vi "Main.vi"() -> ()   [LabVIEW 2021]
doc: "This template is for the Queued Message Handler design pattern.\n\nThe Event Handling Loop generates messages based on user interface actions.\n\nThe Message Handling Loop processes messages generated by the Event Handling Loop, or by other messages. The messages are string values, so new messages can be added easily to the Message Cases case structure in the Message Handling Loop. Each message cluster can also provide an optional value for Message Data, which is a variant that can be converted to whatever message-specific data is required."
uses:
  Czytaj RS/Biblioteki/Statyw/Sending Params.ctl
  controls/UI Data.ctl
  controls/STAV Data.ctl
  Czytaj RS/Biblioteki/Statyw/STAV CommandList.ctl
  support/Message Queue/Enqueue Message (Single).vi
  <vilib>/Utility/error.llb/Error Cluster From Error Code.vi
  <vilib>/ErrorRing/Error Ring.xnode
  support/Message Queue/Message Queue.lvlib
  support/User Event - Stop/User Event - Stop.lvlib
  Czytaj RS/Biblioteki/Statyw/STAV lib.lvlib
panel:
  out "str command":string
  out "String 2":string
  out "String":string
  out "Display <Replace Me>":string
  in  "Exit":bool
  in  "Tab Control":T1(tab)
  in  "STAV com port":refnum<visa-resource-name>="COM6"
  in  "Sending Params (set before RUN)":T2={"[s]peed"=FALSE, "[p]osition"=TRUE, "[f]orce"=TRUE, "p[e]ak force"=FALSE, "pe[a]k distance"=FALSE, "[t]ravel"=FALSE, "[m]s"=TRUE, "[c]ycle no"=FALSE, "step [n]o"=FALSE, "[d]uration"=FALSE, "p[r]ofile position"=FALSE, "[h]old time"=FALSE}
  in  "Sending Interval":i32=500 min=1 max=10000 step=1
  in  "StopSending":bool
  in  "Velocity":i32=30
  in  "Position":dbl
  in  "HomePos":bool
  in  "Start Sending":bool
  in  "Clear 2":bool
  out "Log 2":string
  in  "Clear":bool
  out "Log":string
  in  "Do Something <Replace Me>":bool
  in  "Do Something Else <Replace Me>":bool
  # "These controls have associated \"Value Changed\" events configured in the Event Structure on the diagram.\n\nReplace them (and reconfigure the Event Structure) with the controls you need for your application."
  # "This template is for the Queued Message Handler design pattern.\n\nSee the block diagram for more information on how to use this template."
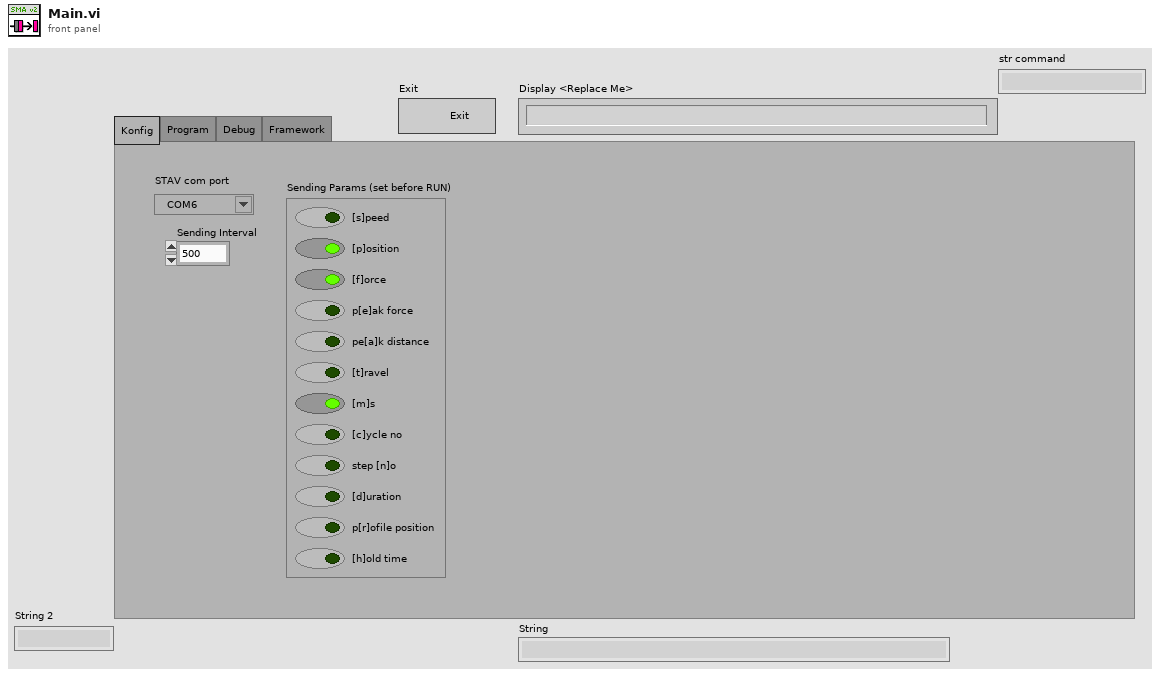
[diagram p1: front panel]
types:
  T1 = enum32{"Konfig", "Program", "Debug", "Framework"}
  T2 = typedef "STAV lib.lvlib/Sending Params.ctl" = cluster{"[s]peed":bool, "[p]osition":bool, "[f]orce":bool, "p[e]ak force":bool, "pe[a]k distance":bool, "[t]ravel":bool, "[m]s":bool, "[c]ycle no":bool, "step [n]o":bool, "[d]uration":bool, "p[r]ofile position":bool, "[h]old time":bool}
  T3 = typedef "STAV Data.ctl" = cluster{"STAV ref":refnum<visa-resource-name>}
  T4 = typedef "UI Data.ctl" = cluster{"Boolean <Replace Me>":bool, "String <Replace Me>":string, "Numeric <Replace Me>":dbl, "Do Something Ref":refnum<vi>, "Do Something Else Ref":refnum<vi>, "Data Display Ref":refnum<vi>, "Exit Button Ref":refnum<vi>}
  T5 = typedef "Message Queue.lvlib/All Message Queues.ctl" = cluster{"UI":refnum<queue>, "Display":refnum<queue>, "Stav":refnum<queue>, "DAQ":refnum<queue>}
  T6 = typedef "STAV lib.lvlib/STAV CommandList.ctl" = enum16{"StartSending (0)", "StopSending(0)", "FindHomePos(0)", "SetSendingConfig(2)", "GetSendingConfig(0)", "SetPosition(2)", "SetSpeed(2)", "GetSpeed(0)", "GetPosition(0)", "GetForce(0)", "GetPeak(0)", "GetPeakDistance(0)", "GetTravelDistance(0)", "ResetTravelDistance(0)", "GetCycleNo(0)", "GetStepNo(0)", "GetDuration(0)", "GetProfilePosition(0)", "GetHoldTime(0)", "Stop(0)", "StartAndSend(0)", "Start(0)", "Reset(0)", "GetActiveProfile(0)", "SetActiveProfile(2)", "GetProfileCnt(1)", "GetMaxStepCnt(1)", "GetStepCnt(2)", "GetProfileIndex(2)", "SetProfile(3)", "SetStep(3+params)", "GetProfile(2)", "GetStep(3)", "SetProfile(2+params)", ""}
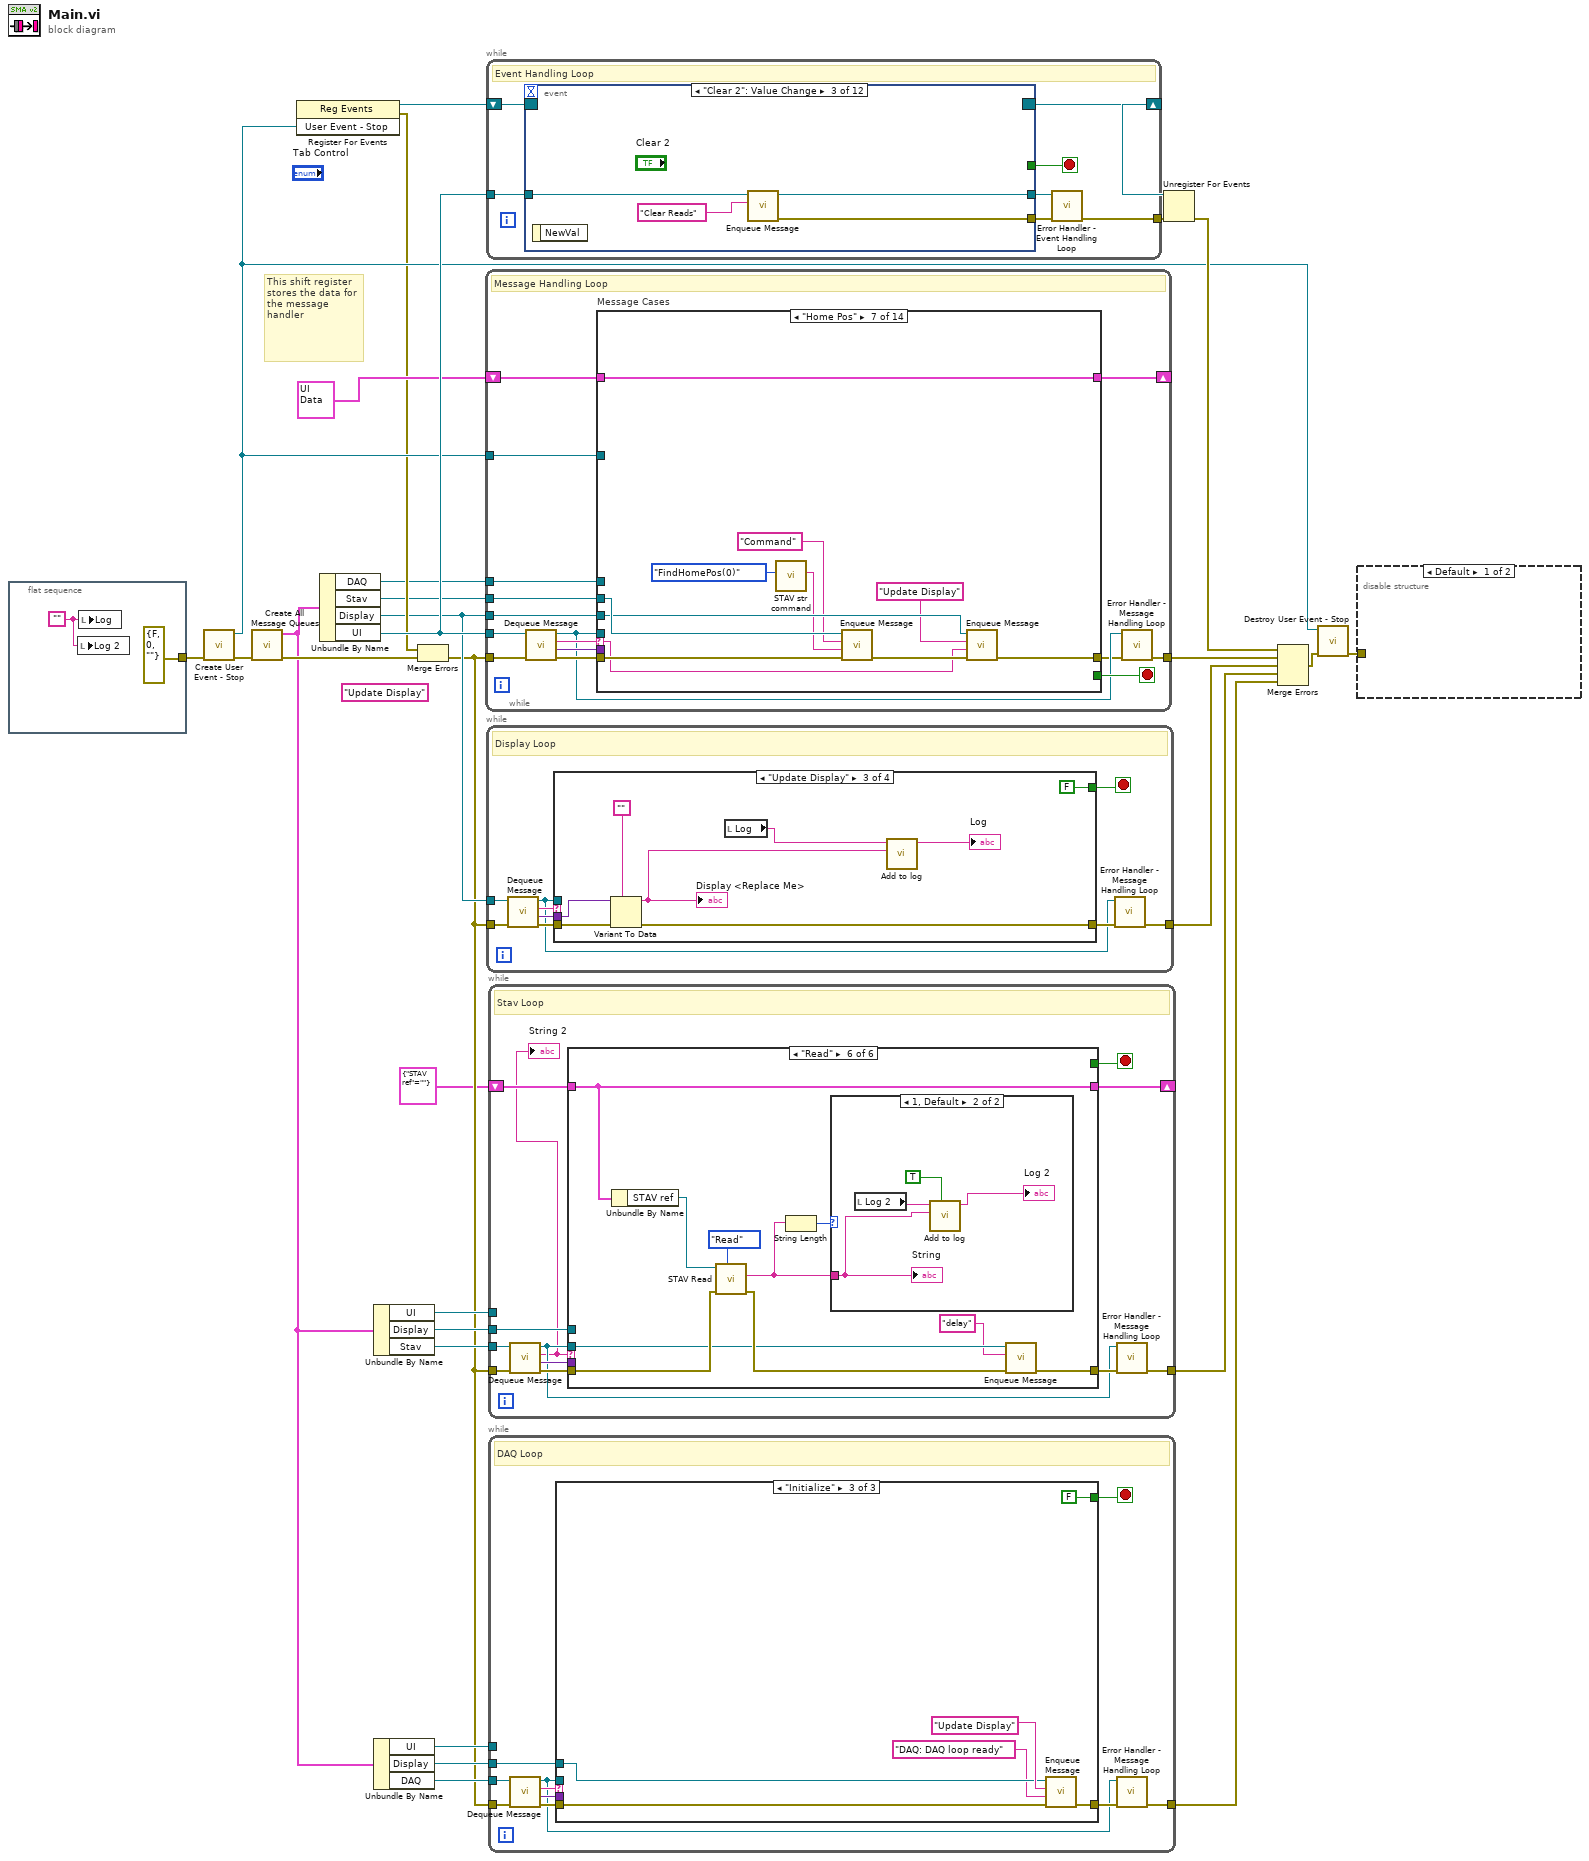
[diagram p0: block diagram]
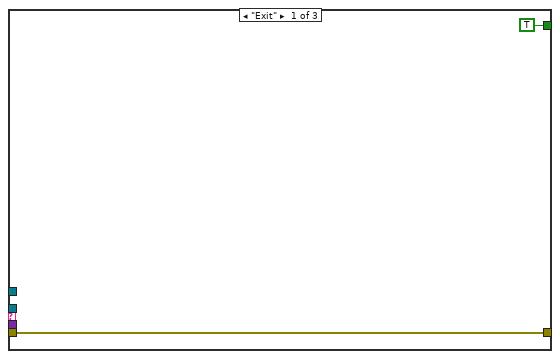
[diagram p2: hidden frame]
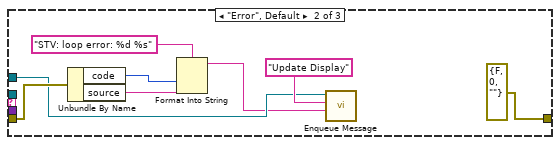
[diagram p3: hidden frame]
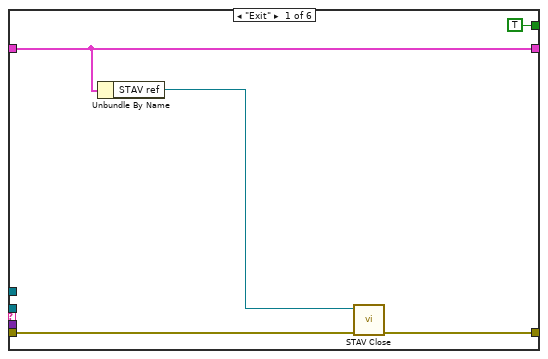
[diagram p4: hidden frame]
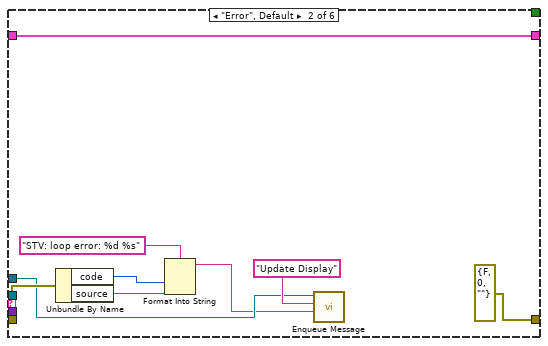
[diagram p5: hidden frame]
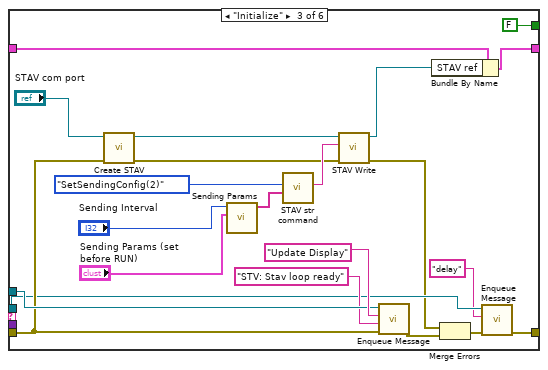
[diagram p6: hidden frame]
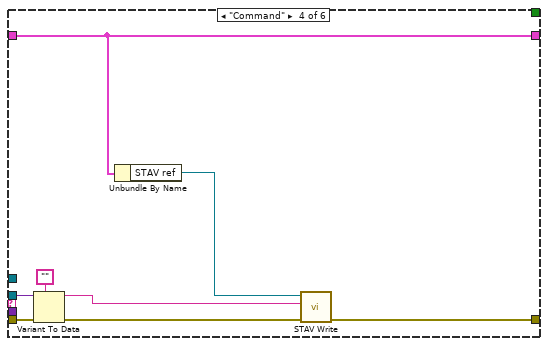
[diagram p7: hidden frame]
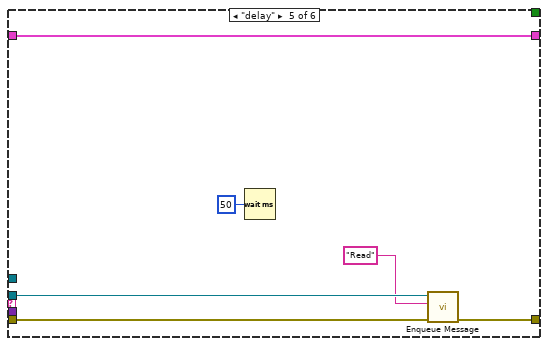
[diagram p8: hidden frame]
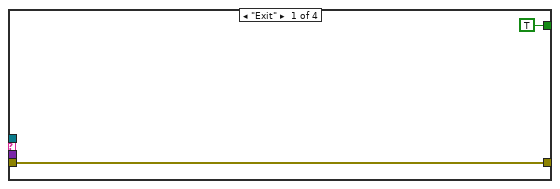
[diagram p10: hidden frame]
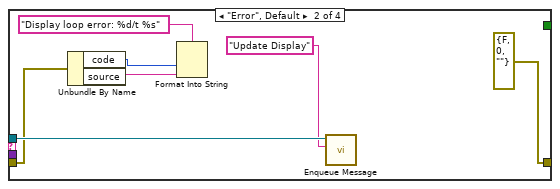
[diagram p11: hidden frame]
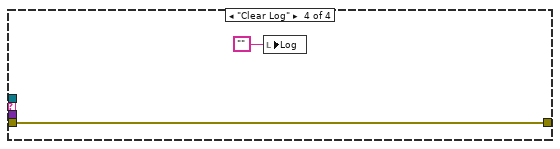
[diagram p12: hidden frame]
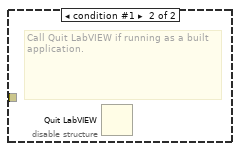
[diagram p13: hidden frame]
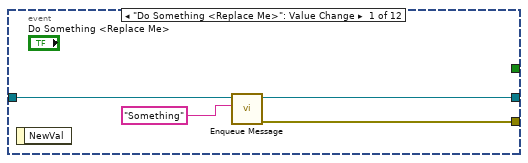
[diagram p14: hidden frame]
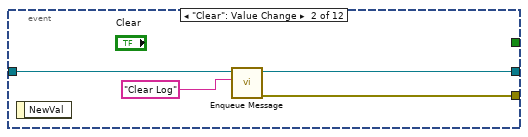
[diagram p15: hidden frame]
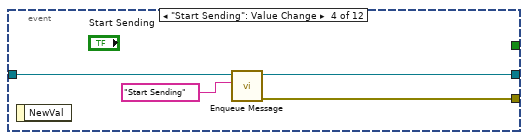
[diagram p16: hidden frame]
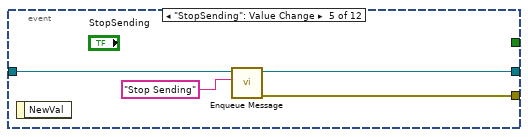
[diagram p17: hidden frame]
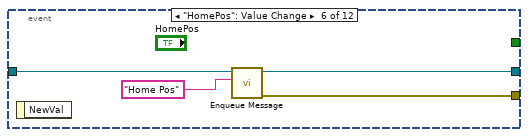
[diagram p18: hidden frame]
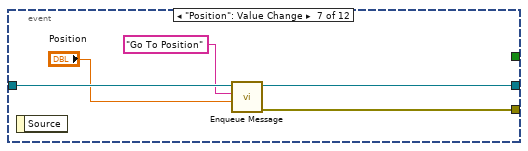
[diagram p19: hidden frame]
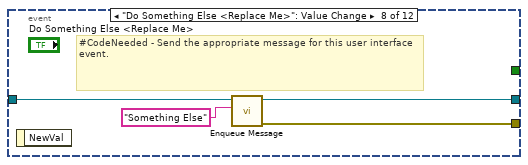
[diagram p20: hidden frame]
diagram:
  (unwired) "Update Display" ("Message")
  # "This shift register stores the data for the message handler"
  n1 = flat-sequence {
    tunnel: [errorcluster {"status"=FALSE, "code"=0, "source"=""} ("error constant")] -> w11
    frame #0 {
      w30 = ""
      n2 = local write "Log 2"(w30) -> ()
      n3 = local write "Log"(w30) -> ()
    }
  }
  n4 = call "Create User Event - Stop.vi"("error in (no error)"=w11) -> ("error out"=w26:errorcluster, "User Event - Stop"=w18:refnum<user-event>)  [unwired: 9 in]
  n5 = call "Create All Message Queues.vi"("error in (no error)"=w26) -> ("error out"=w29:errorcluster, "Message Queues out"=w4:T5)  [unwired: 9 in]
  n6 = register-events(w18) -> (reference out=w19:refnum<event-registration>, error out=w17:errorcluster)  [unwired: 2 in]
  n7 = Unbundle By Name(w4) -> ("DAQ"=w14:refnum<queue>, "Stav"=w15:refnum<queue>, "Display"=w16:refnum<queue>, "UI"=w27:refnum<queue>)
  n8 = Unbundle By Name(w4) -> ("UI"=w8:refnum<queue>, "Display"=w12:refnum<queue>, "Stav"=w13:refnum<queue>)
  n9 = Unbundle By Name(w4) -> ("UI"=w7:refnum<queue>, "Display"=w6:refnum<queue>, "DAQ"=w5:refnum<queue>)
  n10 = Merge Errors(w17, w29) -> (w2:errorcluster)
  n11 = while {
    tunnel: w27 -> [w38]
    shift-right: [w45] -> _
    shift-left: T4 {"Boolean <Replace Me>"=FALSE, "String <Replace Me>"="", "Numeric <Replace Me>"=0.0, "Do Something Ref"=refnum, "Do Something Else Ref"=refnum, "Data Display Ref"=refnum, "Exit Button Ref"=refnum} ("Data Cluster") -> [w46]
    tunnel: w18 -> [w43]
    tunnel: w2 -> [w42]
    tunnel: [w36] -> w28
    tunnel: w16 -> [w34]
    tunnel: w15 -> [w33]
    tunnel: w14 -> [w32]
    stop <- w44 stop-if-true
    # "Message Handling Loop"
    n12 = call "Dequeue Message.vi"("error in (no error)"=w42, "Message Queue"=w38) -> ("error out"=w41:errorcluster, "Message Data"=w39:variant, "Message"=w40:string, "dup Message Queue"=w37:refnum<queue>)  [unwired: 6 in]
    n13 = case "Message Cases" shown="\"Home Pos\"" w40 {
      selector: w40 -> [_ _ _ _ w81 w92 w103 w121 w129 _ _ _ w151 w171]
      tunnel: w37 -> [_ _ _ _ _ _ _ _ _ _ w142 _ w170 _]
      tunnel: w41 -> [w55 w61 w68 w77 w87 w98 w109 w115 w131 w138 w146 w149 w164 _]
      tunnel: [w56 w62 w69 w71 w84 w95 w106 w124 w130 w137 w144 w147 w167 w172] -> w35
      tunnel: w46 -> [w54 w63 w70 w76 w88 w99 w110 w127 w132 w139 w145 w148 w169 w173]
      tunnel: [w53 w63 w70 w76 w88 w99 w110 w127 w132 w139 w145 w148 w169 w173] -> w45
      tunnel: [_ _ _ _ _ _ _ _ _ _ _ _ TRUE _] -> w44
      tunnel: w39 -> [_ _ _ w75 _ _ _ w113 _ _ _ _ w161 _]
      tunnel: w43 -> [_ _ _ _ _ _ _ _ _ _ _ _ w166 _]
      tunnel: w34 -> [w47 w57 w64 _ w83 w94 w105 w123 w128 w136 _ _ w159 _]
      tunnel: w33 -> [_ _ _ _ w86 w97 w108 w126 _ _ _ _ w154 _]
      tunnel: w32 -> [_ _ _ _ _ _ _ _ _ _ _ _ w150 _]
      frame "Initialize" {
        w50 = "MHL: Program Ready" ("Initial Message")
        # "Initialize - All initialization work should take place in this message, since other loops can potentially enqueue messages that execute immediately after this one."
        n14 = control-ref of="Do Something <Replace Me>"() -> (w48:refnum<vi>)
        n15 = control-ref of="Do Something Else <Replace Me>"() -> (w49:refnum<vi>)
        n16 = control-ref of="Exit"() -> (w52:refnum<vi>)
        n17 = Bundle By Name(cluster=w54, "Do Something Ref"=w48, "Do Something Else Ref"=w49, "Exit Button Ref"=w52, "String <Replace Me>"=w50) -> (w53:T4)
        n18 = call-poly "Enqueue Message.vi"("error in (no error)"=w55, "Message Data"=w50, "Message"="Update Display", "Message Queue"=w47) -> ("error out"=w56:errorcluster)  [unwired: 6 in, 1 out]
      }
      frame "Something" {
        # "Send string to \"Update Display\" message"
        # "#CodeNeeded - Perform whatever actions correspond to the \"Something\" message."
        # "Something - Replace this message with functionality for your own application."
        n19 = call-poly "Enqueue Message.vi"("error in (no error)"=w61, "Message Data"="\"Do Something\" button pressed" ("\"Do Something\" button pressed"), "Message"="Update Display", "Message Queue"=w57) -> ("error out"=w60:errorcluster)  [unwired: 6 in, 1 out]
        n20 = Merge Errors(w60) -> (w62:errorcluster)
      }
      frame "Something Else" {
        # "Send string to \"Update Display\" message"
        # "#CodeNeeded - Perform whatever actions correspond to the \"Something Else\" message."
        # "Something Else - Replace this message with functionality for your own application."
        n21 = call-poly "Enqueue Message.vi"("error in (no error)"=w68, "Message Data"="\"Do Something Else\" button pressed" ("\"Do Something Else\" button pressed"), "Message"="Update Display", "Message Queue"=w64) -> ("error out"=w67:errorcluster)  [unwired: 6 in, 1 out]
        n22 = Merge Errors(w67) -> (w69:errorcluster)
      }
      frame "Error" {
        # "#CodeRecommended - If you ever change the name of this \"Error\" message, you'll need to update the name in the Check Loop Error.vi as well."
        # "#CodeRecommended - Consider creating a system for logging errors in some way. These errors are for notification purposes only. Handling of specific errors should be performed in the message frames that generated the error."
        # "Error - Display an error dialog. This message is sent by the \"Error Handler\" VIs at the end of other loops in this application."
        n23 = Variant To Data(error in=w77, type=errorcluster {"status"=FALSE, "code"=0, "source"=""} ("error constant"), Variant=w75) -> (data=w73:errorcluster, error out=w72:errorcluster)
        n24 = call <vilib>:"Simple Error Handler.vi"("error in (no error)"=w73) -> ()  [unwired: 4 in, 5 out]
        n25 = Merge Errors(w72) -> (w71:errorcluster)
      }
      frame "Start Sending" {
        n26 = call "STAV str command.vi"("Command"=STAV_CommandList."StartSending (0)") -> ("str command"=w79:string)  [unwired: 9 in, 1 out]
        n27 = call-poly "Enqueue Message.vi"("error in (no error)"=w87, "Message Data"=w79, "Message"="Command", "Message Queue"=w86) -> ("error out"=w85:errorcluster)  [unwired: 6 in, 1 out]
        n28 = call-poly "Enqueue Message.vi"("error in (no error)"=w85, "Message Data"=w81, "Message"="Update Display", "Message Queue"=w83) -> ("error out"=w84:errorcluster)  [unwired: 6 in, 1 out]
      }
      frame "Stop Sending" {
        n29 = call "STAV str command.vi"("Command"=STAV_CommandList."StopSending(0)") -> ("str command"=w90:string)  [unwired: 9 in, 1 out]
        n30 = call-poly "Enqueue Message.vi"("error in (no error)"=w98, "Message Data"=w90, "Message"="Command", "Message Queue"=w97) -> ("error out"=w96:errorcluster)  [unwired: 6 in, 1 out]
        n31 = call-poly "Enqueue Message.vi"("error in (no error)"=w96, "Message Data"=w92, "Message"="Update Display", "Message Queue"=w94) -> ("error out"=w95:errorcluster)  [unwired: 6 in, 1 out]
      }
      frame "Home Pos" {
        n32 = call "STAV str command.vi"("Command"=STAV_CommandList."FindHomePos(0)") -> ("str command"=w101:string)  [unwired: 9 in, 1 out]
        n33 = call-poly "Enqueue Message.vi"("error in (no error)"=w109, "Message Data"=w101, "Message"="Command", "Message Queue"=w108) -> ("error out"=w107:errorcluster)  [unwired: 6 in, 1 out]
        n34 = call-poly "Enqueue Message.vi"("error in (no error)"=w107, "Message Data"=w103, "Message"="Update Display", "Message Queue"=w105) -> ("error out"=w106:errorcluster)  [unwired: 6 in, 1 out]
      }
      frame "Go To Position" {
        n35 = Variant To Data(error in=w115, type=0.0, Variant=w113) -> (data=w111:dbl, error out=w114:errorcluster)
        n36 = call "Position Attributes.vi"("Speed"="Velocity", "Position"=w111) -> ("array"=w117:string[])  [unwired: 8 in, 1 out]
        n37 = call "STAV str command.vi"("Params"=w117, "Command"=STAV_CommandList."SetPosition(2)") -> ("str command"=w119:string)  [unwired: 8 in, 1 out]
        "str command" <- w119
        n38 = call-poly "Enqueue Message.vi"("error in (no error)"=w114, "Message Data"=w119, "Message"="Command", "Message Queue"=w126) -> ("error out"=w125:errorcluster)  [unwired: 6 in, 1 out]
        n39 = call-poly "Enqueue Message.vi"("error in (no error)"=w125, "Message Data"=w121, "Message"="Update Display", "Message Queue"=w123) -> ("error out"=w124:errorcluster)  [unwired: 6 in, 1 out]
      }
      frame "Clear Log" {
        n40 = call-poly "Enqueue Message.vi"("error in (no error)"=w131, "Message"=w129, "Message Queue"=w128) -> ("error out"=w130:errorcluster)  [unwired: 7 in, 1 out]
      }
      frame "Clear Reads" {
        n41 = call-poly "Enqueue Message.vi"("error in (no error)"=w138, "Message Data"="MHL: Clear Reads" ("Message"), "Message"="Update Display", "Message Queue"=w136) -> ("error out"=w137:errorcluster)  [unwired: 6 in, 1 out]
        n42 = local write "Log 2"("") -> ()
      }
      frame "Confirm Quit" {
        # "#CodeNeeded - If you want to provide an \"Are you sure\" dialog (or some other notification) before the application exits, place that code here. This message is typically sent from a Panel Close? event."
        # "Confirm Quit - Message that can confirm whether or not the user wants to exit the application."
        n43 = call-poly "Enqueue Message.vi"("Priority Message? (F)"=TRUE, "error in (no error)"=w146, "Message"="Exit", "Message Queue"=w142) -> ("error out"=w143:errorcluster)  [unwired: 6 in, 1 out]
        n44 = Merge Errors(w143) -> (w144:errorcluster)
      }
      frame "---Copy This Frame---" {
        # "Duplicate this frame when creating new messages.  Change this comment in the duplicated frame to describe this message."
        n45 = Merge Errors(w149) -> (w147:errorcluster)
      }
      frame "Exit" {
        # "Stop the VI"
        # "#CodeNeeded - Add any required cleanup code here. Note that if 'Exit' was called as a result of an error, an error dialog will be displayed. Add any custom error handling for an 'Exit' condition here as well."
        # "Exit - Exit the application."
        n46 = Variant To Data(type=errorcluster {"status"=FALSE, "code"=0, "source"=""} ("error constant"), Variant=w161) -> (data=w162:errorcluster)  [unwired: 1 in, 1 out]
        n47 = Release Queue(queue=w170, error in (no error)=w164) -> (error out=w160:errorcluster)  [unwired: 1 in, 2 out]
        n48 = call <vilib>:"Simple Error Handler.vi"("error in (no error)"=w162) -> ()  [unwired: 4 in, 5 out]
        n49 = call-poly "Enqueue Message.vi"("error in (no error)"=w160, "Message Data"=w151, "Message"="Update Display", "Message Queue"=w159) -> ("error out"=w156:errorcluster, "dup Message Queue"=w157:refnum<queue>)  [unwired: 6 in]
        n50 = call-poly "Enqueue Message.vi"("error in (no error)"=w156, "Message"=w151, "Message Queue"=w157) -> ("error out"=w155:errorcluster)  [unwired: 7 in, 1 out]
        n51 = call "Fire User Event - Stop.vi"("User Event - Stop"=w166) -> ("error out"=w165:errorcluster)  [unwired: 10 in]
        n52 = call-poly "Enqueue Message.vi"("error in (no error)"=w155, "Message"=w151, "Message Queue"=w154) -> ("error out"=w153:errorcluster)  [unwired: 7 in, 1 out]
        n53 = call-poly "Enqueue Message.vi"("error in (no error)"=w153, "Message"=w151, "Message Queue"=w150) -> ("error out"=w152:errorcluster)  [unwired: 7 in, 1 out]
        n54 = Merge Errors(w165, w152) -> (w167:errorcluster)
      }
      frame Default {
        # "'Default' case only runs if there is a message that isn't defined in any of the other cases.  Output a programming error."
        n55 = xnode "Error Ring"("parameter 0"=w171) -> ("error out"=w172:errorcluster)
      }
    }
    n56 = call "Error Handler - Message Handling Loop.vi"("error in (no error)"=w35, "Message Queue"=w37) -> ("dup error in"=w36:errorcluster)  [unwired: 8 in, 1 out]
  }
  n57 = while {
    tunnel: w27 -> [w187]
    shift-right: [w185] -> w23
    shift-left: w19 -> [w186]
    tunnel: [w181] -> w20
    stop <- w183 stop-if-true
    # "Event Handling Loop"
    n58 = event shown="[2] \"Clear 2\": Value Change" {
      selector: w186 -> [_ _ _ _ _ _ _ _ _ _ _ _]
      dyn-events: [_ _ _ _ _ _ _ _ _ _ _ _] -> w185
      timeout: _ -> [_ _ _ _ _ _ _ _ _ _ _ _]
      tunnel: [_ _ _ _ _ _ _ _ _ _ _ TRUE ("Discard?")] -> w183
      tunnel: w187 -> [w191 w195 w199 w203 w207 w211 w216 w220 w225 w227 w232 w234]
      tunnel: [w188 w192 w196 w200 w204 w208 w213 w217 w224 _ w231 _] -> w184
      tunnel: [w190 w194 w198 w202 w206 w210 w215 w219 w223 w227 w230 w234] -> w182
      event "Do Something <Replace Me>": Value Change {
        n59 = event-data() -> ()  [unwired: 1 in, 1 out]
        n60 = call-poly "Enqueue Message.vi"("Message"="Something", "Message Queue"=w191) -> ("error out"=w188:errorcluster, "dup Message Queue"=w190:refnum<queue>)  [unwired: 8 in]
      }
      event "Clear": Value Change {
        n61 = event-data() -> ()  [unwired: 1 in, 1 out]
        n62 = call-poly "Enqueue Message.vi"("Message"="Clear Log", "Message Queue"=w195) -> ("error out"=w192:errorcluster, "dup Message Queue"=w194:refnum<queue>)  [unwired: 8 in]
      }
      event "Clear 2": Value Change {
        n63 = event-data() -> ()  [unwired: 1 in, 1 out]
        n64 = call-poly "Enqueue Message.vi"("Message"="Clear Reads", "Message Queue"=w199) -> ("error out"=w196:errorcluster, "dup Message Queue"=w198:refnum<queue>)  [unwired: 8 in]
      }
      event "Start Sending": Value Change {
        n65 = event-data() -> ()  [unwired: 1 in, 1 out]
        n66 = call-poly "Enqueue Message.vi"("Message"="Start Sending", "Message Queue"=w203) -> ("error out"=w200:errorcluster, "dup Message Queue"=w202:refnum<queue>)  [unwired: 8 in]
      }
      event "StopSending": Value Change {
        n67 = event-data() -> ()  [unwired: 1 in, 1 out]
        n68 = call-poly "Enqueue Message.vi"("Message"="Stop Sending", "Message Queue"=w207) -> ("error out"=w204:errorcluster, "dup Message Queue"=w206:refnum<queue>)  [unwired: 8 in]
      }
      event "HomePos": Value Change {
        n69 = event-data() -> ()  [unwired: 1 in, 1 out]
        n70 = call-poly "Enqueue Message.vi"("Message"="Home Pos", "Message Queue"=w211) -> ("error out"=w208:errorcluster, "dup Message Queue"=w210:refnum<queue>)  [unwired: 8 in]
      }
      event "Position": Value Change {
        n71 = event-data() -> ()  [unwired: 1 in, 1 out]
        n72 = call-poly "Enqueue Message.vi"("Message Data"="Position", "Message"="Go To Position", "Message Queue"=w216) -> ("error out"=w213:errorcluster, "dup Message Queue"=w215:refnum<queue>)  [unwired: 7 in]
      }
      event "Do Something Else <Replace Me>": Value Change {
        # "#CodeNeeded - Send the appropriate message for this user interface event."
        n73 = event-data() -> ()  [unwired: 1 in, 1 out]
        n74 = call-poly "Enqueue Message.vi"("Message"="Something Else", "Message Queue"=w220) -> ("error out"=w217:errorcluster, "dup Message Queue"=w219:refnum<queue>)  [unwired: 8 in]
      }
      event Panel Close? {
        # "Send the 'Confirm Quit' message if the user closes the panel of the VI. Discard the event so the 'Confirm Quit' message has a chance to run."
        n75 = event-data() -> ()  [unwired: 1 in, 1 out]
        n76 = call-poly "Enqueue Message.vi"("Priority Message? (F)"=TRUE, "Message"="Confirm Quit", "Message Queue"=w225) -> ("error out"=w224:errorcluster, "dup Message Queue"=w223:refnum<queue>)  [unwired: 7 in]
        n77 = event-data("Discard?"=TRUE) -> ()  [unwired: 1 in, 1 out]
      }
      event Application Instance Close {
        # "#CodeRecommended - When a project closes, all VIs within that project are aborted and leave memory. However, any code placed in this event frame is guaranteed to run to completion, so add any cleanup code that absolutely must happen here."
        n78 = event-data() -> ()  [unwired: 1 in, 1 out]
      }
      event "Exit": Value Change {
        n79 = event-data() -> ()  [unwired: 1 in, 1 out]
        n80 = call-poly "Enqueue Message.vi"("Priority Message? (F)"=TRUE, "Message"="Exit", "Message Queue"=w232) -> ("error out"=w231:errorcluster, "dup Message Queue"=w230:refnum<queue>)  [unwired: 7 in]
      }
      event User Event {
        (unwired) "\"Exit\" button pressed" ("VI Stopped")
        # "The Message Handling Loop processed an \"Exit\" message, which fired this event to stop the Event Handling Loop."
        n81 = event-data() -> ()  [unwired: 1 in, 1 out]
      }
    }
    n82 = call "Error Handler - Event Handling Loop.vi"("error in (no error)"=w184, "Message Queue"=w182) -> ("dup error in"=w181:errorcluster)  [unwired: 8 in, 1 out]
  }
  n83 = while {
    tunnel: w16 -> [w243]
    tunnel: w2 -> [w242]
    tunnel: [w237] -> w10
    stop <- w236 stop-if-true
    # "Display Loop"
    n84 = call "Dequeue Message.vi"("error in (no error)"=w242, "Message Queue"=w243) -> ("error out"=w241:errorcluster, "Message Data"=w239:variant, "Message"=w240:string, "dup Message Queue"=w235:refnum<queue>)  [unwired: 6 in]
    n85 = case shown="\"Update Display\"" w240 {
      tunnel: w241 -> [w244 w248 w258 w262]
      tunnel: w239 -> [_ _ w257 _]
      tunnel: [w244 errorcluster {"status"=FALSE, "code"=0, "source"=""} ("error out") w256 w262] -> w238
      tunnel: [TRUE _ FALSE _] -> w236
      tunnel: w235 -> [_ w251 _ _]
      frame "Exit" {
      }
      frame "Error", Default {
        n86 = Unbundle By Name(w248) -> ("code"=w247:i32, "source"=w246:string)
        n87 = Format Into String(format string="Display loop error: %d/t %s", w247, w246) -> ()  [unwired: 2 in, 2 out]
        n88 = call-poly "Enqueue Message.vi"("Message"="Update Display", "Message Queue"=w251) -> ()  [unwired: 8 in, 2 out]
      }
      frame "Update Display" {
        n89 = Variant To Data(error in=w258, type="", Variant=w257) -> (data=w254:string, error out=w256:errorcluster)
        "Display <Replace Me>" <- w254
        n90 = local read "Log"() -> (w253:string)
        n91 = call "Add to log.vi"("String in"=w254, "Log"=w253) -> ("String out"=→"Log":string)  [unwired: 9 in]
      }
      frame "Clear Log" {
        n92 = local write "Log"("") -> ()
      }
    }
    n93 = call "Error Handler - Message Handling Loop.vi"("error in (no error)"=w238, "Message Queue"=w235) -> ("dup error in"=w237:errorcluster)  [unwired: 8 in, 1 out]
  }
  n94 = while {
    tunnel: w13 -> [w274]
    tunnel: w2 -> [w273]
    tunnel: [w269] -> w9
    tunnel: w12 -> [w266]
    tunnel: w8 -> [_]
    shift-right: [w264] -> _
    shift-left: T3 {"STAV ref"=""} -> [w265]
    stop <- w268 stop-if-true
    # "Stav Loop"
    n95 = call "Dequeue Message.vi"("error in (no error)"=w273, "Message Queue"=w274) -> ("error out"=w272:errorcluster, "Message Data"=w271:variant, "Message"=w263:string, "dup Message Queue"=w267:refnum<queue>)  [unwired: 6 in]
    "String 2" <- w263
    n96 = case shown="\"Read\"" w263 {
      tunnel: w272 -> [w278 w285 w305 w314 w322 w334]
      tunnel: w271 -> [_ _ _ w313 _ _]
      tunnel: [w276 errorcluster {"status"=FALSE, "code"=0, "source"=""} ("error out") w293 w316 w323 w331] -> w270
      tunnel: [TRUE _ FALSE _ _ _] -> w268
      tunnel: w267 -> [_ _ w292 _ w321 w329]
      tunnel: w266 -> [_ w282 w307 _ _ _]
      tunnel: w265 -> [w277 w280 w303 w318 w324 w333]
      tunnel: [w277 w280 w302 w318 w324 w333] -> w264
      frame "Exit" {
        n97 = Unbundle By Name(w277) -> ("STAV ref"=w275:refnum<visa-resource-name>)
        n98 = call "STAV Close.vi"("error in (no error)"=w278, "STAV ref in"=w275) -> ("error out"=w276:errorcluster)  [unwired: 9 in]
      }
      frame "Error", Default {
        n99 = Unbundle By Name(w285) -> ("code"=w284:i32, "source"=w283:string)
        n100 = Format Into String(format string="STV: loop error: %d %s", w284, w283) -> (resulting string=w281:string)  [unwired: 2 in, 1 out]
        n101 = call-poly "Enqueue Message.vi"("Message Data"=w281, "Message"="Update Display", "Message Queue"=w282) -> ()  [unwired: 7 in, 2 out]
      }
      frame "Initialize" {
        n102 = call "Create STAV.vi"("error in (no error)"=w305, "STAV com port"="STAV com port") -> ("error out"=w298:errorcluster, "STAV ref out"=w301:refnum<visa-resource-name>)  [unwired: 8 in]
        n103 = call "Sending Params.vi"("Sending Params"="Sending Params (set before RUN)", "Interval (100)"="Sending Interval") -> ("params array out"=w296:string[])  [unwired: 7 in, 2 out]
        n104 = call "STAV str command.vi"("Params"=w296, "Command"=STAV_CommandList."SetSendingConfig(2)") -> ("str command"=w299:string)  [unwired: 8 in, 1 out]
        n105 = call "STAV Write.vi"("error in (no error)"=w298, "Command"=w299, "STAV ref in"=w301) -> ("error out"=w289:errorcluster, "STAV ref out"=w290:refnum<visa-resource-name>)  [unwired: 7 in]
        n106 = call-poly "Enqueue Message.vi"("error in (no error)"=w305, "Message Data"="STV: Stav loop ready" ("Message"), "Message"="Update Display", "Message Queue"=w307) -> ("error out"=w309:errorcluster)  [unwired: 6 in, 1 out]
        n107 = Bundle By Name(cluster=w303, "STAV ref"=w290) -> (w302:T3)
        n108 = Merge Errors(w289, w309) -> (w294:errorcluster)
        n109 = call-poly "Enqueue Message.vi"("error in (no error)"=w294, "Message"="delay", "Message Queue"=w292) -> ("error out"=w293:errorcluster)  [unwired: 7 in, 1 out]
      }
      frame "Command" {
        n110 = Variant To Data(error in=w314, type="", Variant=w313) -> (data=w311:string, error out=w312:errorcluster)
        n111 = Unbundle By Name(w318) -> ("STAV ref"=w317:refnum<visa-resource-name>)
        n112 = call "STAV Write.vi"("error in (no error)"=w312, "Command"=w311, "STAV ref in"=w317) -> ("error out"=w316:errorcluster)  [unwired: 7 in, 1 out]
      }
      frame "delay" {
        n113 = Wait (ms)(milliseconds to wait=u32 50) -> ()  [unwired: 1 out]
        n114 = call-poly "Enqueue Message.vi"("error in (no error)"=w322, "Message"="Read", "Message Queue"=w321) -> ("error out"=w323:errorcluster)  [unwired: 7 in, 1 out]
      }
      frame "Read" {
        n115 = Unbundle By Name(w333) -> ("STAV ref"=w332:refnum<visa-resource-name>)
        n116 = call "STAV Read.vi"("Action (Read)"=enum16{"Read", "Init"}."Read", "error in (no error)"=w334, "STAV ref in"=w332) -> ("error out"=w330:errorcluster, "String"=w325:string)  [unwired: 5 in, 2 out]
        n117 = String Length(string=w325) -> (length=w326:i32)
        n118 = case shown="1, Default" w326 {
          tunnel: w325 -> [_ w338]
          frame 0 {
          }
          frame 1, Default {
            n119 = local read "Log 2"() -> (w337:string)
            n120 = call "Add to log.vi"("Rewerse"=TRUE, "String in"=w338, "Log"=w337) -> ("String out"=→"Log 2":string)  [unwired: 8 in]
            "String" <- w338
          }
        }
        n121 = call-poly "Enqueue Message.vi"("error in (no error)"=w330, "Message"="delay", "Message Queue"=w329) -> ("error out"=w331:errorcluster)  [unwired: 7 in, 1 out]
      }
    }
    n122 = call "Error Handler - Message Handling Loop.vi"("error in (no error)"=w270, "Message Queue"=w267) -> ("dup error in"=w269:errorcluster)  [unwired: 8 in, 1 out]
  }
  n123 = while {
    tunnel: w5 -> [w348]
    tunnel: w2 -> [w347]
    tunnel: [w342] -> w3
    tunnel: w6 -> [w339]
    tunnel: w7 -> [_]
    stop <- w341 stop-if-true
    # "DAQ Loop"
    n124 = call "Dequeue Message.vi"("error in (no error)"=w347, "Message Queue"=w348) -> ("error out"=w346:errorcluster, "Message Data"=w344:variant, "Message"=w345:string, "dup Message Queue"=w340:refnum<queue>)  [unwired: 6 in]
    n125 = case shown="\"Initialize\"" w345 {
      tunnel: w346 -> [w349 w355 w362]
      tunnel: w344 -> [_ _ _]
      tunnel: [w349 errorcluster {"status"=FALSE, "code"=0, "source"=""} ("error out") w363] -> w343
      tunnel: [TRUE _ FALSE] -> w341
      tunnel: w340 -> [_ _ _]
      tunnel: w339 -> [_ w352 w360]
      frame "Exit" {
      }
      frame "Error", Default {
        n126 = Unbundle By Name(w355) -> ("code"=w354:i32, "source"=w353:string)
        n127 = Format Into String(format string="STV: loop error: %d %s", w354, w353) -> (resulting string=w351:string)  [unwired: 2 in, 1 out]
        n128 = call-poly "Enqueue Message.vi"("Message Data"=w351, "Message"="Update Display", "Message Queue"=w352) -> ()  [unwired: 7 in, 2 out]
      }
      frame "Initialize" {
        n129 = call-poly "Enqueue Message.vi"("error in (no error)"=w362, "Message Data"="DAQ: DAQ loop ready" ("Message"), "Message"="Update Display", "Message Queue"=w360) -> ("error out"=w363:errorcluster)  [unwired: 6 in, 1 out]
      }
    }
    n130 = call "Error Handler - Message Handling Loop.vi"("error in (no error)"=w343, "Message Queue"=w340) -> ("dup error in"=w342:errorcluster)  [unwired: 8 in, 1 out]
  }
  n131 = Unregister For Events(event registration refnum=w23, error in=w20) -> (error out=w24:errorcluster)
  n132 = Merge Errors(w24, w28, w10, w9, w3) -> (w25:errorcluster)
  n133 = call "Destroy User Event - Stop.vi"("error in (no error)"=w25, "User Event - Stop"=w18) -> ("error out"=w21:errorcluster)  [unwired: 9 in]
  n134 = disable-structure shown="Default" {
    disable-tunnel: w21 -> [_ _]
    frame condition #0 (active) {
    }
    frame condition #1 {
      # "Call Quit LabVIEW if running as a built application."
      n135 = Quit LabVIEW() -> ()  [unwired: 1 in]
    }
  }
